vi "global_str.vi"() -> ()   [LabVIEW 2019]
panel:
  in  "字符串":string
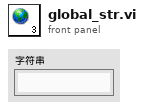
[diagram p1: front panel]
diagram:
